vi "SetUpMotor.vi"(8 "Error In":errorcluster, 10 "Serial Number":string="27004535", 11 "KCubeDCServo in":refnum<k24>) -> (0 "Error Out":errorcluster, 3 "KCubeDCServo out":refnum<k24>)   [LabVIEW 2018, in "Thorlabs.lvlib" / "Thorlabs.lvclass"]
doc: "This VI sets the settings on the Motor Device that is being used.\n\nCreator: Slade Jeppesen\nCreated: 09/29/20"
uses:
  Thorlabs.lvclass
  C:/AME Test Engineering/LabVIEW/PPLs/Axis/DLLs/ThorLabs.MotionControl.KCube.DCServoCLI.dll
  PPLs/Axis/DLLs/ThorLabs.MotionControl.KCube.DCServoCLI.dll
  C:/AME Test Engineering/LabVIEW/PPLs/Axis/DLLs/Thorlabs.MotionControl.GenericMotorCLI.dll
  PPLs/Axis/DLLs/Thorlabs.MotionControl.GenericMotorCLI.dll
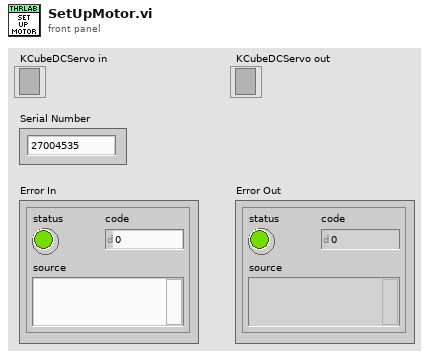
[diagram p1: front panel]
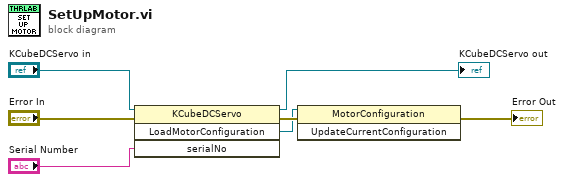
[diagram p0: block diagram]
diagram:
  n1 = invoke class="KCubeDCServo" method="LoadMotorConfiguration"(reference="KCubeDCServo in", error in="Error In", "serialNo"="Serial Number") -> (reference out=→"KCubeDCServo out":refnum<k24>, error out=w2:errorcluster, "LoadMotorConfiguration"=w1:refnum<k24>)  [unwired: 1 in, 1 out]
  n2 = invoke class="MotorConfiguration" method="UpdateCurrentConfiguration"(reference=w1, error in=w2) -> (error out=→"Error Out":errorcluster)  [unwired: 1 in, 2 out]
